vi "load correction table.vi"(8 "error in (no error)":errorcluster, 10 "namefile":string, 11 "id":i32) -> (0 "error out":errorcluster, 2 "function return":i32, 3 "id out":i32)   [LabVIEW 2012, in "libximc.lvlib"]
doc: "result_t XIMC_API load_correction_table(device_t* id, const char* namefile);"
uses:
  libximc.lvlib
  libximc.dll
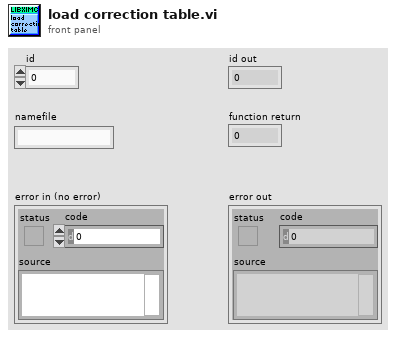
[diagram p1: front panel]
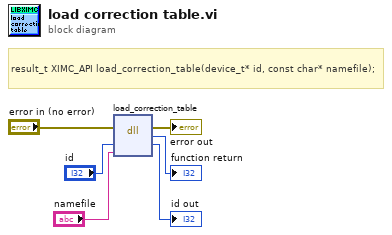
[diagram p0: block diagram]
diagram:
  # "result_t XIMC_API load_correction_table(device_t* id, const char* namefile);"
  n1 = dll-call lib="E:/labview-2.12.1-Labview_12.0/ximcLVx32/libximc.*" fn="load_correction_table"(error in="error in (no error)", "id"="id", "namefile"="namefile") -> (error out=→"error out":errorcluster, →"function return":i32, "id"=→"id out":i32)  [unwired: 3 in, 1 out]
